vi "rad_Merge AppImage Properties.vi"(0 "RAD property":string, 2 "SysCfg property":string) -> (4 "New Property":string)   [LabVIEW 2014]
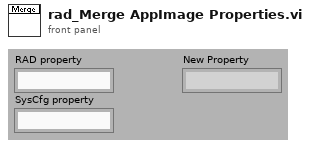
[diagram p1: front panel]
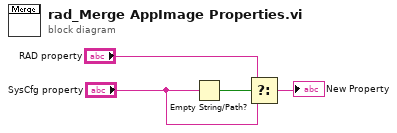
[diagram p0: block diagram]
diagram:
  n1 = Empty String/Path?(string/path="SysCfg property") -> (empty?=w4:bool)
  n2 = Select(t="RAD property", s=w4, f="SysCfg property") -> (s? t:f=→"New Property":string)
